vi "Init.vi"(10 "Transport Type":T1) -> (0 "Error out":errorcluster, 2 "Transport out":refnum<class "Transport.lvclass">)   [LabVIEW 2025, in "jettl.lvlib" / "Transport.lvlib"]
uses:
  Transport.lvlib
  Actor/Transport Type.ctl
  Transport/Transport.lvclass
  Event Transport/Event Transport.lvclass
  C:/git/jettl/src/jettl/jettl/Transport/Transport/Transport.lvclass
  Actor/Actor.lvlib
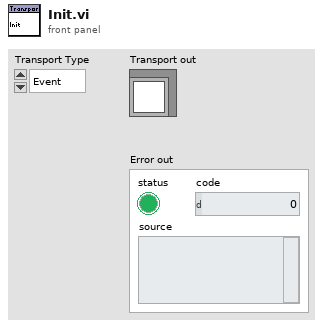
[diagram p1: front panel]
types:
  T1 = typedef "jettl.lvlib/Actor.lvlib/Transport Type.ctl" = enum16{"Event", "Queue"}
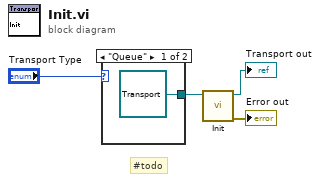
[diagram p0: block diagram]
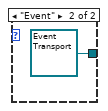
[diagram p2: hidden frame]
diagram:
  # "#todo"
  n1 = case shown="\"Queue\"" "Transport Type" {
    tunnel: [refnum<class "Transport.lvclass"> refnum ("jettl.lvlib:Transport.lvlib:Transport.lvclass") refnum<class "Event Transport.lvclass"> refnum ("jettl.lvlib:Transport.lvlib:Event Transport.lvclass")] -> w1
    frame "Queue" {
    }
    frame "Event" {
    }
  }
  n2 = call-dynamic "Init.vi"("Transport in"=w1) -> ("Error out"=→"Error out":errorcluster, "Transport out"=→"Transport out":refnum<class "Transport.lvclass">)  [unwired: 9 in]
